vi "AverageOfArray(SubVI).vi"(10 "Array":dbl[](array[numeric])) -> (2 "Average of array":dbl)   [LabVIEW 2014]
doc: "This SubVI finds the average of the elements in an array."
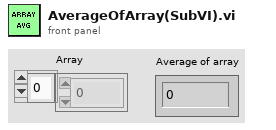
[diagram p1: front panel]
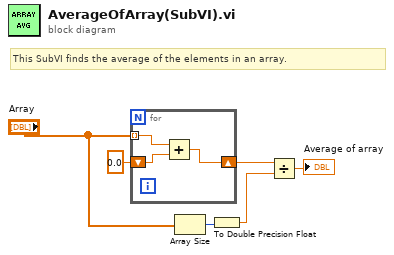
[diagram p0: block diagram]
diagram:
  # "This SubVI finds the average of the elements in an array."
  n1 = for {
    tunnel: "Array" -> [w9] mode=indexing
    shift-right: [w8] -> w6
    shift-left: 0.0 -> [w7]
    n2 = Add(x=w9, y=w7) -> (x+y=w8:dbl)
  }
  n3 = Array Size(array="Array") -> (size(s)=w3:i32)
  n4 = To Double Precision Float(number=w3) -> (double precision float=w2:dbl)
  n5 = Divide(x=w6, y=w2) -> (x/y=→"Average of array":dbl)
